vi "Drive_Loop_Camera_Sensor.vi"(9 "Stable?":bool, 10 "Camera Angle":dbl, 11 "Drive Loop Cluster":T1) -> ()   [LabVIEW 2015]
doc: "Help file written by FRC Team 836 - The RoboBees\n\nThis VI writes a camera angle into the Camera Sensor RT FIFO.\n\nThe RT FIFO has to be initialized using the \"Drive_Loop_Initialize_w_Help\" VI."
uses:
  <userlib>/836-Library/Drive/Drive_Code/Drive_Code_Support/Drive_Code_Bundle.ctl
  <userlib>/836-Library/Drive/Drive_Code/Drive_Code_Support/Sensor_Cluster.ctl
  <userlib>/836-Library/Drive/Drive_Code/Drive_Code_Support/Camera_Cluster.ctl
  <userlib>/836-Library/Drive/Drive_Code/Drive_Code_Support/Drive_Code_Notifier.ctl
  <userlib>/836-Library/Drive/Drive_Code/Drive_Code_Support/Drive_Code_Command.ctl
  <userlib>/836-Library/Drive/Drive_Code/Logging_Data.ctl
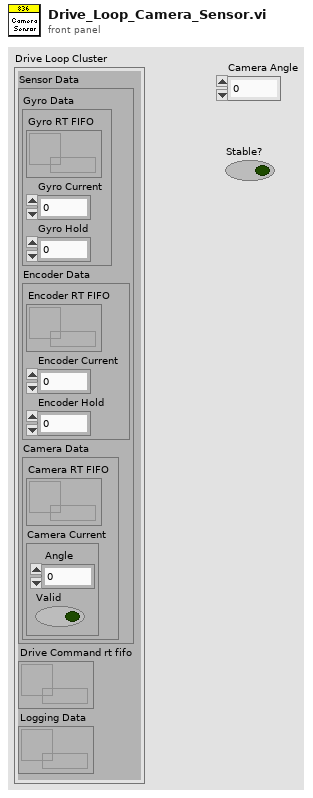
[diagram p1: front panel]
types:
  T1 = typedef "Drive_Code_Bundle.ctl" = cluster{"Sensor Data":T2, "Drive Command rt fifo":refnum<k33>, "Logging Data":refnum<k33>}
  T2 = typedef "Sensor_Cluster.ctl" = cluster{"Gyro Data":cluster{"Gyro RT FIFO":refnum<k33>, "Gyro Current":dbl, "Gyro Hold":dbl}, "Encoder Data":cluster{"Encoder RT FIFO":refnum<k33>, "Encoder Current":dbl, "Encoder Hold":dbl}, "Camera Data":cluster{"Camera RT FIFO":refnum<k33>, "Camera Current":T3}}
  T3 = typedef "Camera_Cluster.ctl" = cluster{" Angle":dbl, "Valid":bool}
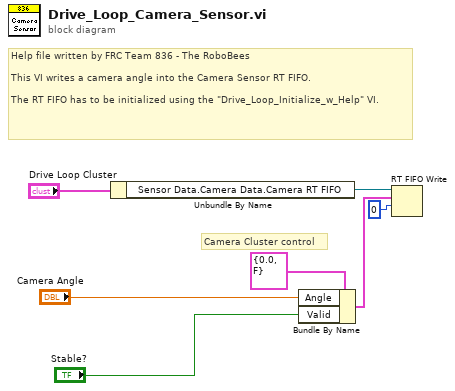
[diagram p0: block diagram]
diagram:
  # "Help file written by FRC Team 836 - The RoboBees\n\nThis VI writes a camera angle into the Camera Sensor RT FIFO.\n\nThe RT FIFO has to be initialized using the \"Drive_Loop_Initialize_w_Help\" VI."
  # "Camera Cluster control"
  n1 = Unbundle By Name("Drive Loop Cluster") -> ("Sensor Data.Camera Data.Camera RT FIFO"=w7:refnum<k33>)
  n2 = Bundle By Name(cluster=T3 {" Angle"=0.0, "Valid"=FALSE}, "Angle"="Camera Angle", "Valid"="Stable?") -> (w4:T3)
  n3 = RT FIFO Write(0:w7, 1:w4, 2:0 ("timeout in ms (0)")) -> ()  [unwired: 2 in, 4 out]
